vi "SEA_CURRENT_CONTROL_REFERENCE_TEST.vi"() -> ()   [LabVIEW 2019]
uses:
  <vilib>/Platform/TimedLoop/XDataNode/timing_clust.ctl
  <vilib>/Platform/TimedLoop/XDataNode/nitl_modes.ctl
  <vilib>/Platform/TimedLoop/XDataNode/wakeup.ctl
  <vilib>/FPGAPlugInAG/sbRIO-9627/niLvFpga_Open_sbRIO-9627.vi
  <vilib>/rvi/interface/common/dynamic/niFpgaDynamicAddResources.vi
  <vilib>/Utility/error.llb/Error Cluster From Error Code.vi
  <vilib>/rvi/errors/niLvFpgaAdjustHostInterfaceError.vi
  <vilib>/FPGAPlugInAG/Dynamic/niLvFpga_Close_Dynamic.vi
  <vilib>/rvi/interface/nirviOpenFPGA/nirviOpenFPGA.xnode
  FPGA Bitfiles/seafinalexperime_FPGATarget_SEALOWERLEVELCON_meT+vsors+U.lvbitx
  SEA_LOWER_LEVEL_CONTROL.vi
  <vilib>/platform/TimedLoop/XDataNode/XDataNode.xnode
  <vilib>/rvi/interface/nirviReadWriteControl/nirviReadWriteControl.xnode
  <vilib>/rvi/interface/nirviCloseFPGA/nirviCloseFPGA.xnode
  NiFpgaLv.dll
  <vilib>/rvi/interface/Simulation/niFpgaSimulationCallBeginRW.vi
  <vilib>/Platform/TimedLoop/XDataNode/XDNodeRunTimeDep.lvlib
panel:
  out "Numeric":u32
  out "Waveform Chart":cluster{sgl, "Filtered Current(M2)":sgl}(graph)
  out "control_ip":sgl
  in  "KpGain":sgl
  in  "Current Offset":sgl
  in  "Amplitude":sgl
  in  "frequency":sgl
  out "motor direction":bool
  in  "stop":bool
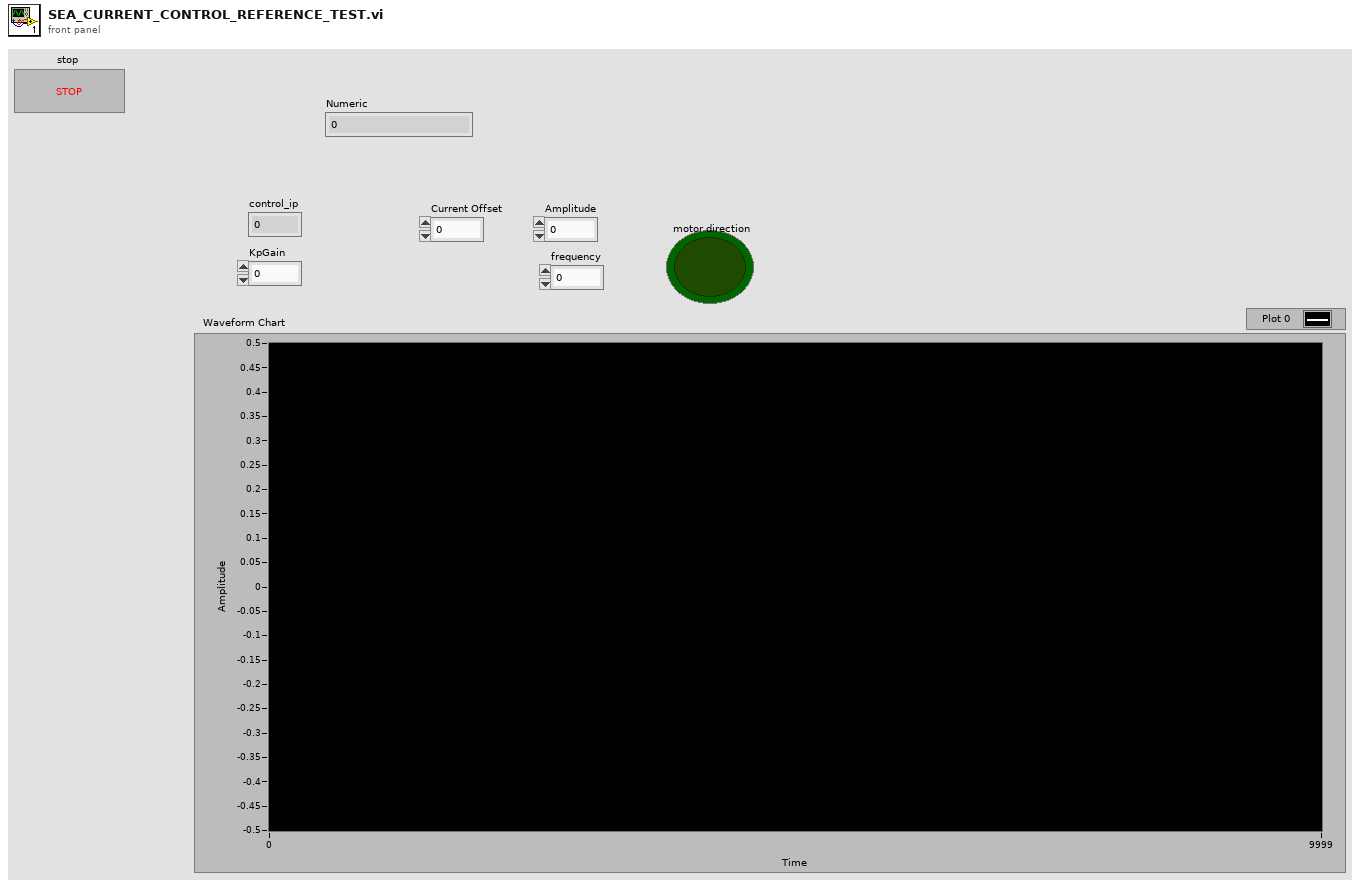
[diagram p1: front panel]
types:
  T1 = typedef "XDNodeRunTimeDep.lvlib/timing_clust.ctl" = cluster{"Expected End [f-1]":u64, "Actual End [f-1]":u64, "Finished Late? [f-1]":bool, "Expected End [i-1]":u64, "Actual End [i-1]":u64, "Finished Late? [i-1]":bool, "Expected Start [i]":u64, "Actual Start [i]":u64, "Expected Start [f]":u64, "Actual Start [f]":u64, "Source Name":string, "Structure Name":string, "Period":i64, "Deadline":i64, "Offset":i64, "Start":i64, "Priority":i32, "Timeout":i32, "Mode":T2, "Wakeup Reason":T3, "Error":errorcluster, "Source Type":string, "Secondary Source Type":string, "Global End Time":u64, "Global Start Time":u64, "Frame Duration":u64, "Iteration Duration":u64, "Assigned CPU":i32, "I/O Scan Engine Mode":u32}
  T2 = typedef "XDNodeRunTimeDep.lvlib/nitl_modes.ctl" = enum32{"No Change", "Process missed periods, maintain original phase", "Discard missed periods, maintain original phase", "Process missed periods, ignore original phase", "Discard missed periods, ignore original phase"}
  T3 = typedef "XDNodeRunTimeDep.lvlib/wakeup.ctl" = enum32{"Normal", "Aborted", "Asynchronous wakeup", "Timing source error", "Timed loop error", "Timeout"}
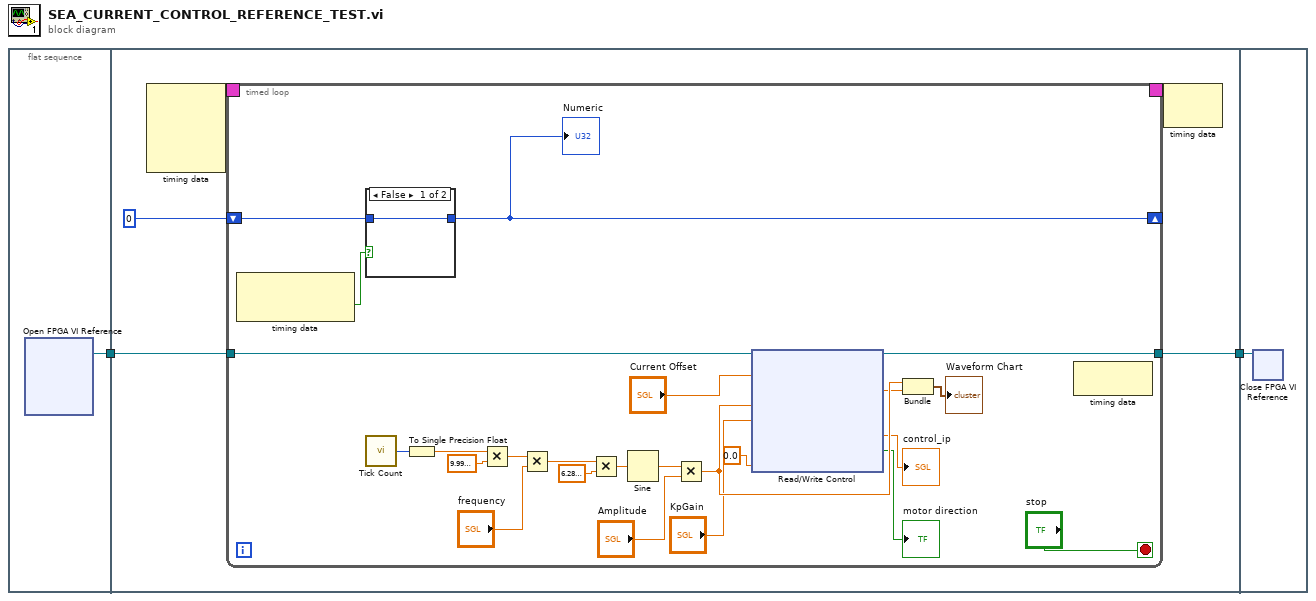
[diagram p0: block diagram]
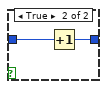
[diagram p2: hidden frame]
diagram:
  n1 = flat-sequence {
    tunnel: [w3] -> w2
    tunnel: w2 -> [w8]
    tunnel: [w7] -> w1
    tunnel: w1 -> [w41]
    frame #0 {
      n2 = xnode "Open FPGA VI Reference"() -> ("FPGA VI Reference Out"=w3:refnum<k20>)  [unwired: 2 in, 1 out]
    }
    frame #1 {
      n3 = node-c288() -> (w6:T1)  [unwired: 4 in]
      n4 = timed-loop {
        tunnel: w8 -> [w19]
        tunnel: [w17] -> w7
        timing: w6 -> [_]
        timing-out: [_] -> w5
        shift-right: [w9] -> _
        shift-left: u32 0 -> [w10]
        stop <- "stop" stop-if-true
        n5 = node-c288() -> (w11:bool)  [unwired: 1 in, 1 out]
        n6 = case shown="False" w11 {
          tunnel: w10 -> [w33 w35]
          tunnel: [w33 w34] -> w9
          frame False {
          }
          frame True {
            n7 = Increment(x=w35) -> (x+1=w34:u32)
          }
        }
        "Numeric" <- w9
        n8 = call "Tick Count"() -> ("Tick Count(uSec)"=w29:u32)
        n9 = To Single Precision Float(number=w29) -> (single precision float=w30:sgl)
        n10 = Multiply(x=w30, y=sgl 1e-06) -> (x*y=w31:sgl)
        n11 = Multiply(x=w31, y="frequency") -> (x*y=w28:sgl)
        n12 = Multiply(x=w28, y=sgl 6.28) -> (x*y=w27:sgl)
        n13 = Sine(x=w27) -> (sin(x)=w26:sgl)
        n14 = Multiply(x=w26, y="Amplitude") -> (x*y=w25:sgl)
        n15 = xnode "Read/Write Control"("FPGA VI Reference In"=w19, "Current Offset"="Current Offset", "reference"=w25, "KpGain"="KpGain", "Tracking zero offset"=sgl 0.0) -> ("FPGA VI Reference Out"=w17:refnum<k20>, "Filtered Current(M2)"=w24:sgl, "control_ip"=→"control_ip":sgl, "motor direction"=→"motor direction":bool)  [unwired: 1 in, 1 out]
        n16 = Bundle(w25, "Filtered Current(M2)"=w24) -> (→"Waveform Chart":cluster{sgl, "Filtered Current(M2)":sgl})  [unwired: 1 in]
        n17 = node-c288() -> ()  [unwired: 1 in, 1 out]
      }
      n18 = node-c288(w5) -> ()  [unwired: 1 out]
    }
    frame #2 {
      n19 = xnode "Close FPGA VI Reference"("FPGA VI Reference In"=w41) -> ()  [unwired: 1 in, 1 out]
    }
  }
